vi "Get Framed Test Channel Path.vi"(8 "error in (no error)":errorcluster, 11 "Edit Test Channel Model in":refnum<class "Edit Test Channel Model.lvclass">) -> (0 "error out":errorcluster, 2 "Framed Test Channel Path":path, 3 "Edit Test Channel Model out":refnum<class "Edit Test Channel Model.lvclass">)   [LabVIEW 2013, in "Edit Test Channel Model.lvlib" / "Edit Test Channel Model.lvclass"]
uses:
  Edit Test Channel Model.lvclass
  Edit Test Channel Model.lvclass/Edit Test Channel Model.ctl
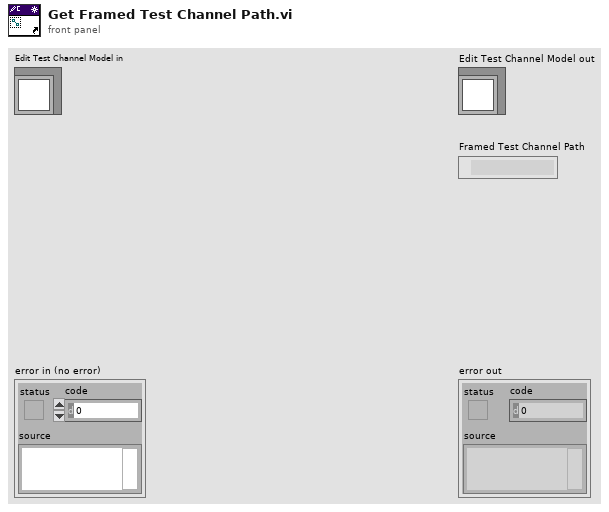
[diagram p1: front panel]
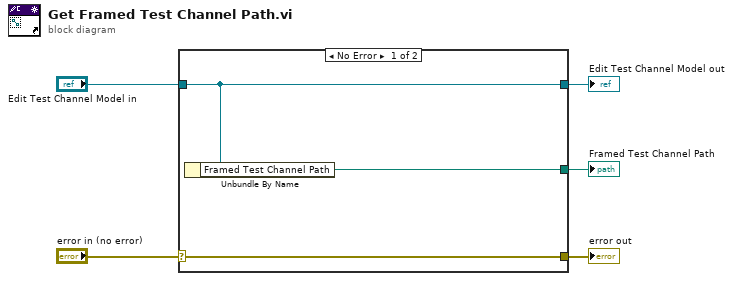
[diagram p0: block diagram]
diagram:
  n1 = case shown="No Error" "error in (no error)" {
    selector: "error in (no error)" -> [w8 w9]
    tunnel: [w8 w9] -> w4
    tunnel: [w7 w10] -> w2
    tunnel: "Edit Test Channel Model in" -> [w7 w10]
    tunnel: [w6 _] -> w1
    frame No Error {
      n2 = Unbundle By Name(w7) -> ("Framed Test Channel Path"=w6:path)
    }
    frame Error {
    }
  }
  "error out" <- w4
  "Edit Test Channel Model out" <- w2
  "Framed Test Channel Path" <- w1
